vi "Read Data.vi"(6 "Sample Count (401)":u32=401, 7 "Format  (0: FDATA)":u16(ring) items=["FDATA", "SDATA", "FMEM", "SMEM", "SDIV"], 8 "Error In (no error)":errorcluster, 9 "Measurement Name (MY_MEAS)":string="MY_MEAS", 10 "Channel (1)":i32=1, 11 "VISA Resource Name":refnum<visa-resource-name>) -> (0 "Error Out":errorcluster, 2 "Data":dbl[](array[numeric]) format="%.15f", 3 "VISA Resource Name Out":refnum<visa-resource-name>)   [LabVIEW 2018, in "Agilent PNA Series.lvlib"]
doc: "This VI reads measurement data in selected format."
uses:
  Agilent PNA Series.lvlib
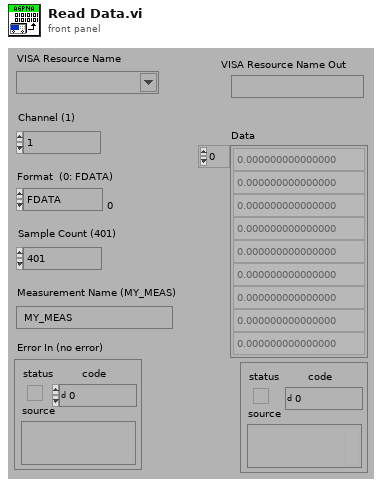
[diagram p1: front panel]
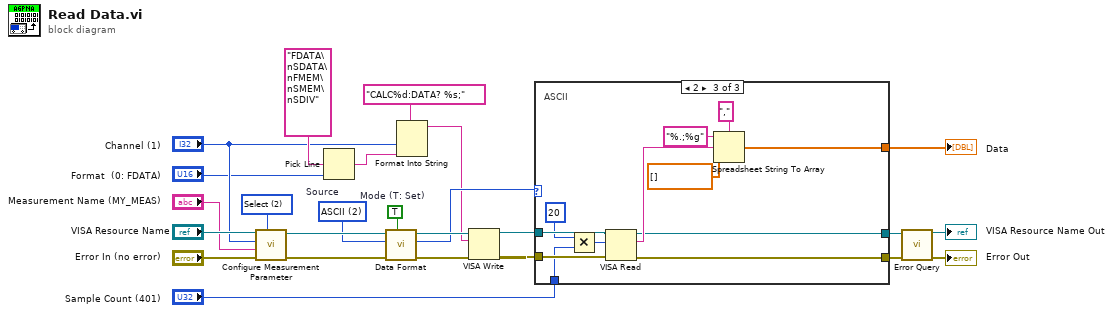
[diagram p0: block diagram]
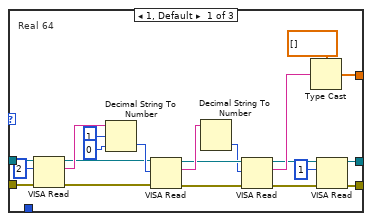
[diagram p2: hidden frame]
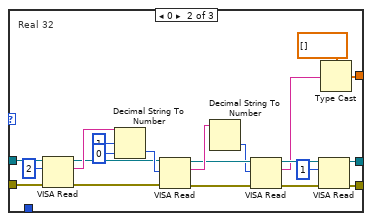
[diagram p3: hidden frame]
diagram:
  w5 = u16 2 items=["Real 32", "Real 64", "ASCII"]  # Source
  w13 = TRUE  # Mode (T: Set)
  w18 = u16 2 items=["Create", "Delete", "Select"] ("Mode (0: Create)")
  n1 = call "Configure Measurement Parameter.vi"("Mode (0: Create)"=w18, "Error In (no error)"="Error In (no error)", "Measurement Name (MY_MEAS)"="Measurement Name (MY_MEAS)", "Channel (1)"="Channel (1)", "VISA Resource Name"="VISA Resource Name") -> ("Error Out"=w6:errorcluster, "VISA Resource Name Out"=w7:refnum<visa-resource-name>)  [unwired: 5 in]
  n2 = Pick Line(multi-line string="FDATA\nSDATA\nFMEM\nSMEM\nSDIV", line index="Format  (0: FDATA)") -> (output string=w23:string)  [unwired: 1 in]
  n3 = call "Data Format.vi"("Mode (T: Set)"=w13, "Error In (no error)"=w6, "Source (0: Real 32)"=w5, "VISA Resource Name"=w7) -> ("Error Out"=w15:errorcluster, "Source"=w14:u16, "VISA Resource Name Out"=w16:refnum<visa-resource-name>)  [unwired: 5 in]
  n4 = Format Into String(format string="CALC%d:DATA? %s;", "Channel (1)", w23) -> (resulting string=w8:string)  [unwired: 2 in, 1 out]
  n5 = VISA Write(VISA resource name=w16, write buffer=w8, error in (no error)=w15) -> (VISA resource name out=w12:refnum<visa-resource-name>, error out=w11:errorcluster)  [unwired: 1 out]
  n6 = case shown="2" w14 {
    tunnel: [w31 w47 w71] -> w9
    tunnel: w12 -> [w46 w57 w76]
    tunnel: w11 -> [w45 w56 w75]
    tunnel: "Sample Count (401)" -> [_ _ w69]
    tunnel: [w26 w51 w73] -> w3
    tunnel: [w27 w52 w72] -> w4
    frame 1, Default {
      # "Real 64"
      n7 = VISA Read(VISA resource name=w46, byte count=u32 2 ("byte count (0)"), error in (no error)=w45) -> (VISA resource name out=w38:refnum<visa-resource-name>, read buffer=w41:string, error out=w39:errorcluster)  [unwired: 1 out]
      n8 = Decimal String To Number(string=w41, offset=1, default (0L)=0) -> (number=w40:i32)  [unwired: 1 out]
      n9 = VISA Read(VISA resource name=w38, byte count=w40, error in (no error)=w39) -> (VISA resource name out=w36:refnum<visa-resource-name>, read buffer=w37:string, error out=w35:errorcluster)  [unwired: 1 out]
      n10 = Decimal String To Number(string=w37) -> (number=w34:i32)  [unwired: 2 in, 1 out]
      n11 = VISA Read(VISA resource name=w36, byte count=w34, error in (no error)=w35) -> (VISA resource name out=w29:refnum<visa-resource-name>, read buffer=w32:string, error out=w28:errorcluster)  [unwired: 1 out]
      n12 = Type Cast(type=dbl[] [], x=w32) -> (*(type *) &x=w31:dbl[])
      n13 = VISA Read(VISA resource name=w29, byte count=u32 1 ("byte count (0)"), error in (no error)=w28) -> (VISA resource name out=w27:refnum<visa-resource-name>, error out=w26:errorcluster)  [unwired: 2 out]
    }
    frame 0 {
      # "Real 32"
      n14 = VISA Read(VISA resource name=w57, byte count=u32 2 ("byte count (0)"), error in (no error)=w56) -> (VISA resource name out=w61:refnum<visa-resource-name>, read buffer=w64:string, error out=w62:errorcluster)  [unwired: 1 out]
      n15 = Decimal String To Number(string=w64, offset=1, default (0L)=0) -> (number=w63:i32)  [unwired: 1 out]
      n16 = VISA Read(VISA resource name=w61, byte count=w63, error in (no error)=w62) -> (VISA resource name out=w59:refnum<visa-resource-name>, read buffer=w60:string, error out=w58:errorcluster)  [unwired: 1 out]
      n17 = Decimal String To Number(string=w60) -> (number=w55:i32)  [unwired: 2 in, 1 out]
      n18 = VISA Read(VISA resource name=w59, byte count=w55, error in (no error)=w58) -> (VISA resource name out=w54:refnum<visa-resource-name>, read buffer=w48:string, error out=w53:errorcluster)  [unwired: 1 out]
      n19 = VISA Read(VISA resource name=w54, byte count=u32 1 ("byte count (0)"), error in (no error)=w53) -> (VISA resource name out=w52:refnum<visa-resource-name>, error out=w51:errorcluster)  [unwired: 2 out]
      n20 = Type Cast(type=sgl[] [], x=w48) -> (*(type *) &x=w47:sgl[])
    }
    frame 2 {
      # "ASCII"
      n21 = Multiply(x=u32 20, y=w69) -> (x*y=w70:u32)
      n22 = VISA Read(VISA resource name=w76, byte count=w70, error in (no error)=w75) -> (VISA resource name out=w72:refnum<visa-resource-name>, read buffer=w74:string, error out=w73:errorcluster)  [unwired: 1 out]
      n23 = Spreadsheet String To Array(delimiter (Tab)=",", format string="%.;%g", spreadsheet string=w74, array type (2D Dbl)=ext[] []) -> (array=w71:ext[])
    }
  }
  "Data" <- w9
  n24 = call "Error Query.vi"("VISA Resource Name"=w4, "error in (no error)"=w3) -> ("VISA Resource Name Out"=→"VISA Resource Name Out":refnum<visa-resource-name>, "error out"=→"Error Out":errorcluster)  [unwired: 10 in, 2 out]
